vi "KUKA youBot Global Value.vi"() -> ()   [LabVIEW 2017, in "NI_Robotics_KUKA youBot Host.lvlib"]
uses:
  <vilib>/robotics/KUKA youBot/NI_Robotics_KUKA youBot Host.lvlib
panel:
  in  "ErrYouBot_MailboxStatus":string[](array[string])=["EtherCAT communication is busy.", "Successfully executed, no error.", "Invalid command.", "Wrong type.", "Configuration EEPROM locked.", "Command not available.", "Parameter is password protected."]
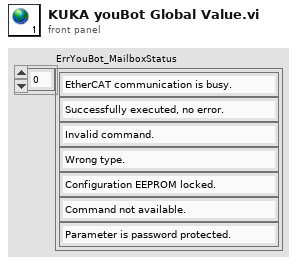
[diagram p1: front panel]
diagram:
